vi "test Properties.vi"(8 "error in (no error)":errorcluster, 11 "TestCase in":refnum<class "Test_Blob.lvclass">) -> (0 "error out":errorcluster, 3 "TestCase out":refnum<class "Test_Blob.lvclass">)   [LabVIEW 2015, in "Test_Blob.lvclass"]
uses:
  Test_Blob.lvclass
  Blob Storage/Blob Type.ctl
  Core/Name Value Pair.ctl
  Global Parameters.vi
  Core/Session/Session.lvclass
  Blob Storage/NI_Azure_Blob.lvlib
  Core/NI_Azure_Core.lvlib
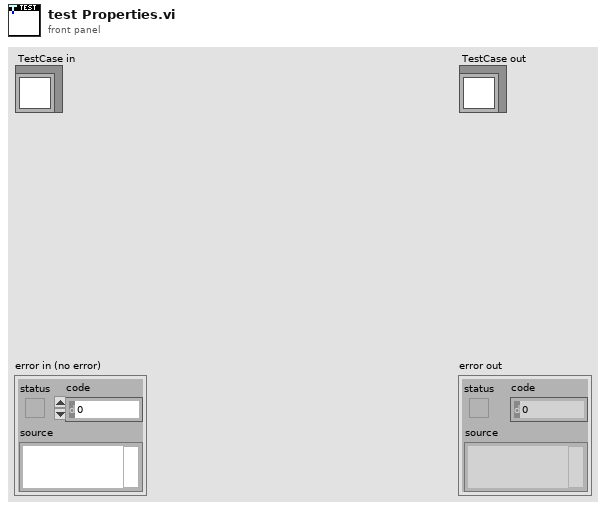
[diagram p1: front panel]
types:
  T1 = typedef "NI_Azure_Core.lvlib/Name Value Pair.ctl" = cluster{"name":string, "value":string}
  T2 = typedef "NI_Azure_Blob.lvlib/Blob Type.ctl" = enum16{"BlockBlob", "PageBlob", "AppendBlob"}
  T3 = typedef "NI_Azure_Core.lvlib/Azure Credentials.ctl" = cluster{"Storage Account Name":string, "Access Key":string}
  T4 = typedef "NI_Azure_Blob.lvlib/Blob Service Properties.ctl" = cluster{"Logging":T5, "Hour metrics":T7, "Minute metrics":T7, "Cors rule":T8, "Default service version":string}
  T5 = typedef "NI_Azure_Blob.lvlib/Logging.ctl" = cluster{"Version":dbl, "Delete":bool, "Read":bool, "Write":bool, "Retention policy":T6}
  T6 = typedef "NI_Azure_Blob.lvlib/Retention Policy.ctl" = cluster{"Enabled":bool, "Days":u32}
  T7 = typedef "NI_Azure_Blob.lvlib/Metrics.ctl" = cluster{"Version":dbl, "Enabled":bool, "Include APIs":bool, "Retention policy":T6}
  T8 = typedef "NI_Azure_Blob.lvlib/Cors Rule.ctl" = cluster{"Allowed origins":string[], "Allowed methods":string[], "Max Age (s)":u32, "Exposed headers":string[], "Allowed headers":string[]}
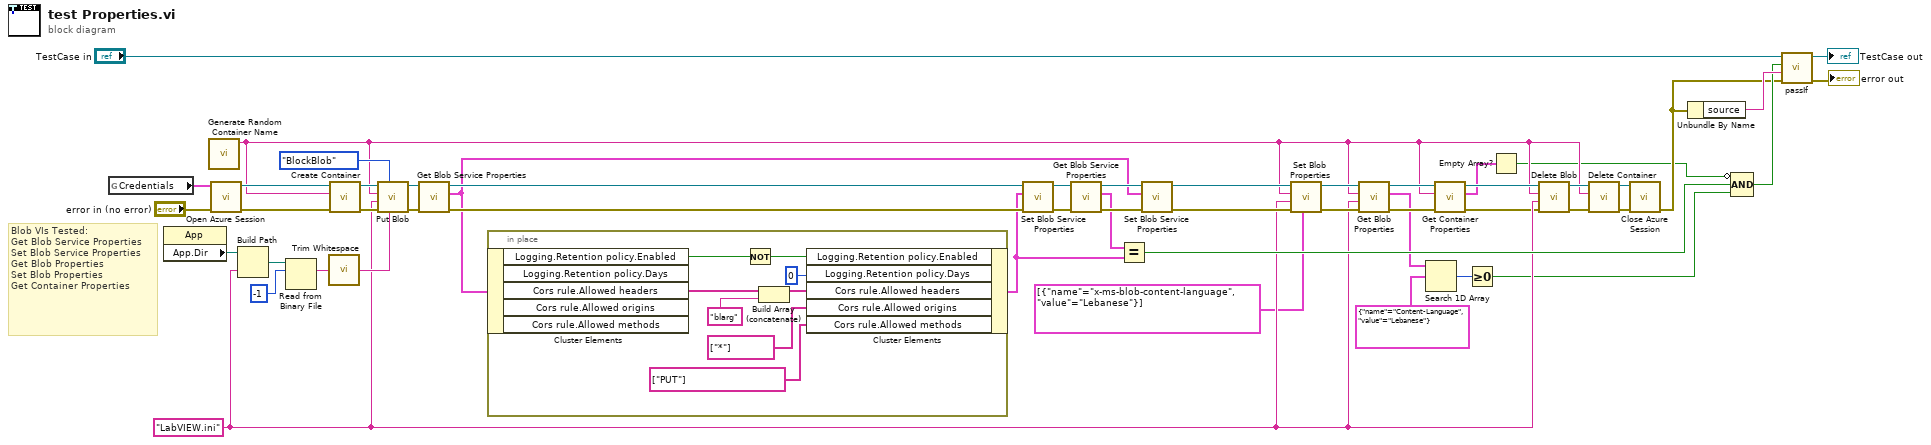
[diagram p0: block diagram]
diagram:
  w12 = "LabVIEW.ini"
  # "Blob VIs Tested:\nGet Blob Service Properties\nSet Blob Service Properties\nGet Blob Properties\nSet Blob Properties\nGet Container Properties"
  n1 = global read "Global Parameters.vi" "Credentials"() -> (w36:T3)
  n2 = property class="App"() -> ("App.Dir"=w47:path)  [unwired: 2 in, 2 out]
  n3 = call "Generate Random Container Name.vi"() -> ("Random Container Name"=w3:string)  [unwired: 11 in]
  n4 = call "Open Azure Session.vi"("error in (no error)"="error in (no error)", "Credentials"=w36) -> ("error out"=w37:errorcluster, "Azure Session"=w33:refnum<class "Session.lvclass">)  [unwired: 8 in]
  n5 = Build Path(base path=w47, name or relative path=w12) -> (appended path=w46:path)
  n6 = Read from Binary File(10:-1 ("count (1)"), 11:w46) -> (2:w41:string)  [unwired: 4 in, 3 out]
  n7 = call <vilib>:"Trim Whitespace.vi"("string"=w41) -> ("trimmed string"=w32:string)  [unwired: 1 in]
  n8 = call "Create Container.vi"("error in (no error)"=w37, "Container"=w3, "Azure Session in"=w33) -> ("error out"=w44:errorcluster, "Azure Session out"=w43:refnum<class "Session.lvclass">)  [unwired: 7 in]
  n9 = call "Put Blob.vi"("Blob Content"=w32, "Blob type"=Blob_Type."BlockBlob", "error in (no error)"=w44, "Blob"=w12, "Container"=w3, "Azure Session in"=w43) -> ("error out"=w42:errorcluster, "Azure Session out"=w27:refnum<class "Session.lvclass">)  [unwired: 4 in]
  n10 = call "Get Blob Service Properties.vi"("error in (no error)"=w42, "Azure Session in"=w27) -> ("error out"=w28:errorcluster, "Blob Service Properties"=w17:T4, "Azure Session out"=w25:refnum<class "Session.lvclass">)  [unwired: 7 in]
  n11 = in-place {
    n12 = in-place-cluster #1(w17) -> ("Logging.Retention policy.Enabled"=w59:bool, "Cors rule.Allowed headers"=w56:string[])  [unwired: 3 out]
    n13 = Not(x=w59) -> (.not. x?=w58:bool)
    n14 = Build Array (concatenate)(w56, "blarg") -> (w55:string[])
    n15 = in-place-cluster #1("Logging.Retention policy.Enabled"=w58, "Logging.Retention policy.Days"=u32 0, "Cors rule.Allowed headers"=w55, "Cors rule.Allowed origins"=string[] ["*"], "Cors rule.Allowed methods"=string[] ["PUT"]) -> (w21:T4)
  }
  n16 = call "Set Blob Service Properties.vi"("error in (no error)"=w28, "Blob Service Properties"=w21, "Azure Session in"=w25) -> ("error out"=w26:errorcluster, "Azure Session out"=w23:refnum<class "Session.lvclass">)  [unwired: 7 in]
  n17 = call "Get Blob Service Properties.vi"("error in (no error)"=w26, "Azure Session in"=w23) -> ("error out"=w24:errorcluster, "Blob Service Properties"=w22:T4, "Azure Session out"=w18:refnum<class "Session.lvclass">)  [unwired: 7 in]
  n18 = Equal?(x=w22, y=w21) -> (x = y?=w20:bool)
  n19 = call "Set Blob Service Properties.vi"("error in (no error)"=w24, "Blob Service Properties"=w17, "Azure Session in"=w18) -> ("error out"=w19:errorcluster, "Azure Session out"=w14:refnum<class "Session.lvclass">)  [unwired: 7 in]
  n20 = call "Set Blob Properties.vi"("Header name-value pairs"=T1[] [{"name"="x-ms-blob-content-language", "value"="Lebanese"}], "error in (no error)"=w19, "Blob"=w12, "Container"=w3, "Azure Session in"=w14) -> ("error out"=w15:errorcluster, "Azure Session out"=w13:refnum<class "Session.lvclass">)  [unwired: 5 in]
  n21 = call "Get Blob Properties.vi"("error in (no error)"=w15, "Blob"=w12, "Container"=w3, "Azure Session in"=w13) -> ("error out"=w16:errorcluster, "Blob Properties"=w10:T1[], "Azure Session out"=w5:refnum<class "Session.lvclass">)  [unwired: 5 in]
  n22 = Search 1D Array(1D array=w10, element=T1 {"name"="Content-Language", "value"="Lebanese"}) -> (index of element=w8:i32)  [unwired: 1 in]
  n23 = call "Get Container Properties.vi"("error in (no error)"=w16, "Container"=w3, "Azure Session in"=w5) -> ("error out"=w6:errorcluster, "Container Properties"=w2:T1[], "Azure Session out"=w4:refnum<class "Session.lvclass">)  [unwired: 6 in]
  n24 = Greater Or Equal To 0?(x=w8) -> (x >= 0?=w7:bool)
  n25 = Empty Array?(array=w2) -> (empty?=w1:bool)
  n26 = call "Delete Blob.vi"("error in (no error)"=w6, "Blob"=w12, "Container"=w3, "Azure Session in"=w4) -> ("error out"=w40:errorcluster, "Azure Session out"=w39:refnum<class "Session.lvclass">)  [unwired: 6 in]
  n27 = call "Delete Container.vi"("error in (no error)"=w40, "Container"=w3, "Azure Session in"=w39) -> ("error out"=w35:errorcluster, "Azure Session out"=w29:refnum<class "Session.lvclass">)  [unwired: 7 in]
  n28 = call "Close Azure Session.vi"("error in (no error)"=w35, "Azure Session"=w29) -> ("error out"=w30:errorcluster)  [unwired: 9 in]
  n29 = Unbundle By Name(w30) -> ("source"=w48:string)
  n30 = Compound Arithmetic op=AND(invert w1, w20, w7) -> (w34:bool)
  n31 = call-dynamic "passIf.vi"("error in (no error)"=w30, "message (\"\")"=w48, "pass"=w34, "TestCase in"="TestCase in") -> ("error out"=→"error out":errorcluster, "TestCase out"=→"TestCase out":refnum<class "Test_Blob.lvclass">)  [unwired: 6 in]
